vi "piecyk_23.vi"(3 "Stop Button":bool, 4 "Desired Temperature °C":i32(knob) min=-20 max=50 step=1 scale=-20.0..50.0, 5 "VISA resource":refnum<visa-resource-name>) -> (0 "Heating ON/OFF":bool, 1 "Temp. Chart":i32(graph), 2 "Current temp °C":dbl(slide) scale=-20.0..50.0 scale format="%#_1p")   [LabVIEW 2024]
doc: "Use this template to build a standard state machine design pattern. Each state executes code and determines which state to transition to. Contrast this design pattern with the User Interface Event Handler pattern, in which code executes in response to user actions. Contrast this design pattern also with the Queued Message Handler pattern, in which each message handling code can queue zero or more new messages.\nNote: This template does not contain the most recent programming guidelines recommended by National Instruments. For a complete, project-based implementation of the Standard State Machine pattern, use the Create Project dialog box instead of this template."
uses:
  piecyk.ctl
  <vilib>/Instr/_visa.llb/VISA Configure Serial Port (Instr).vi
panel:
  out "Temp indicator":string
  # "Time"
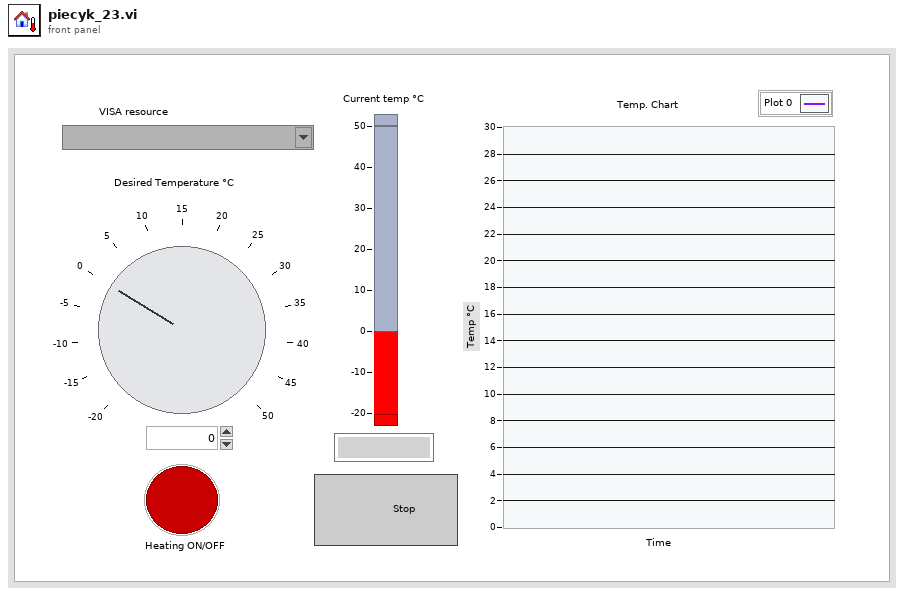
[diagram p1: front panel]
types:
  T1 = typedef "piecyk.ctl" = enum16{"Initialize", "Heating", "Ho Heating", "Stop"}
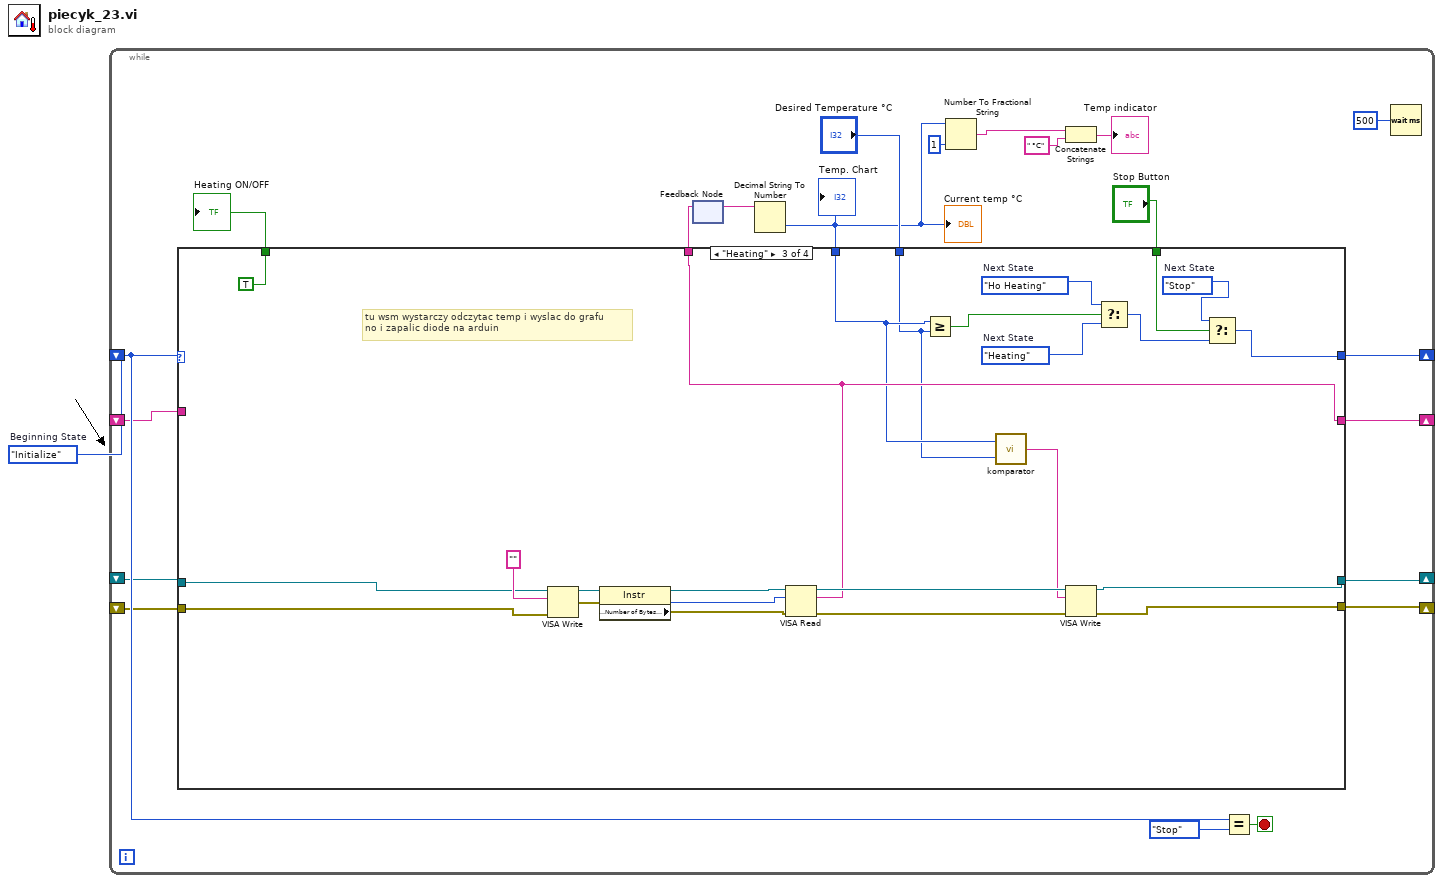
[diagram p0: block diagram]
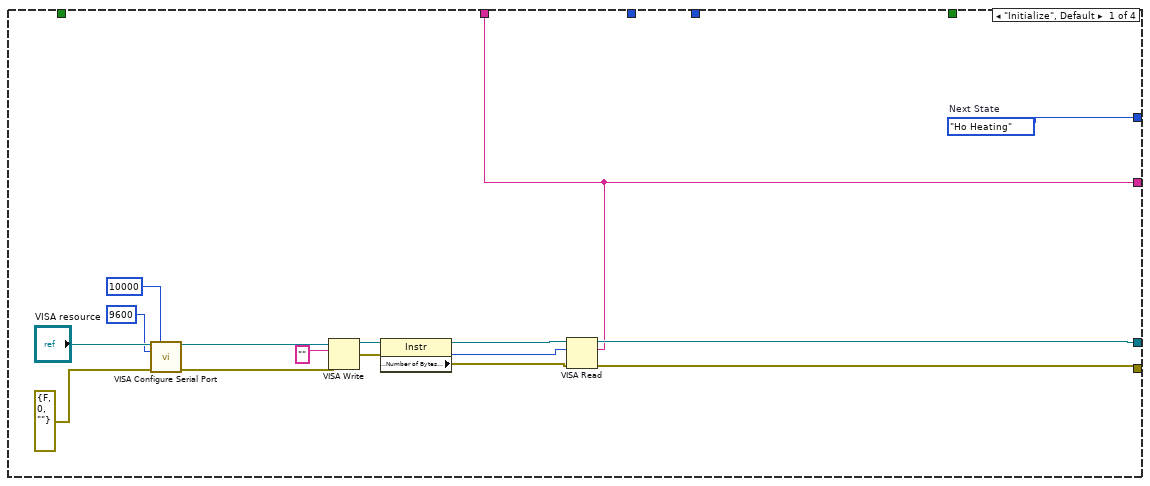
[diagram p2: hidden frame]
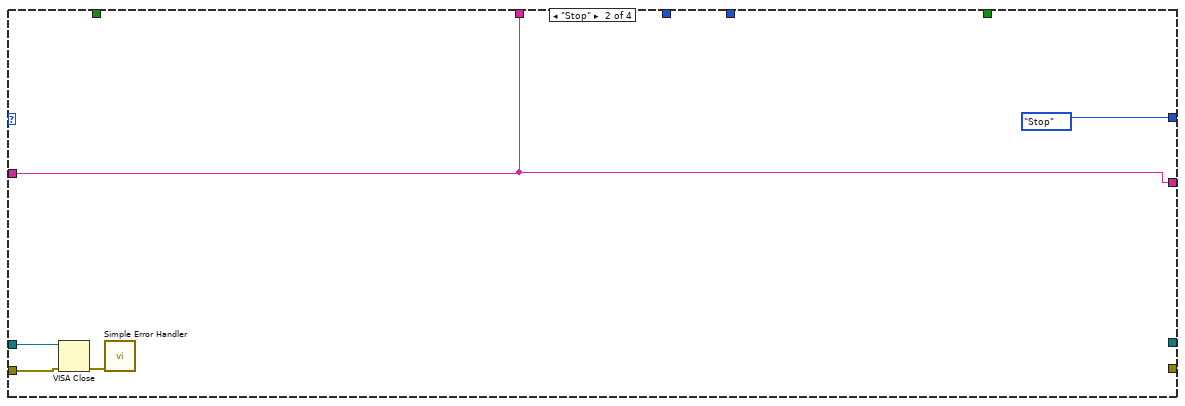
[diagram p3: hidden frame]
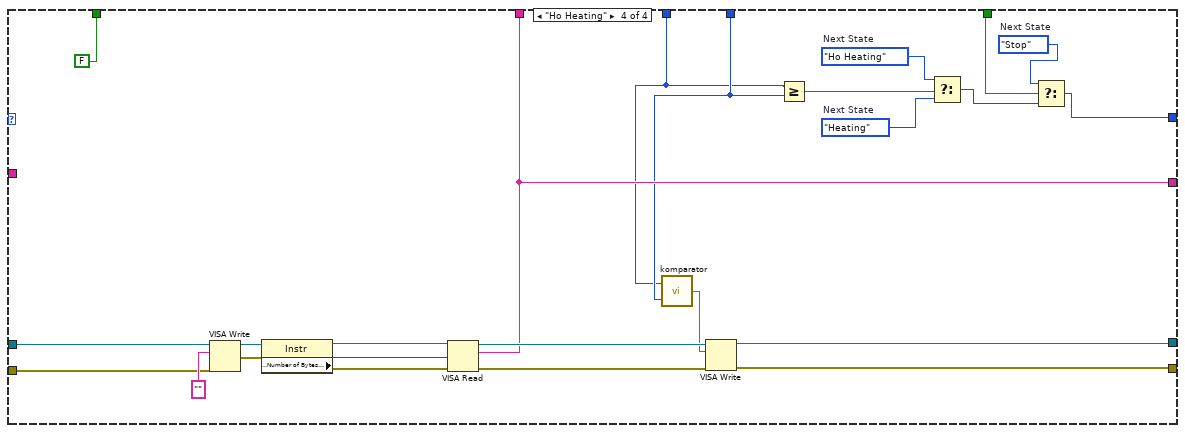
[diagram p4: hidden frame]
diagram:
  w1 = piecyk."Initialize"  # Beginning State
  n1 = while {
    shift-right: [w18] -> _
    shift-left: w1 -> [w20]
    shift-right: [w17] -> _
    shift-left: _ -> [w7]
    shift-right: [w16] -> _
    shift-left: _ -> [w6]
    shift-right: [w3] -> _
    shift-left: _ -> [w2]
    stop <- w22 stop-if-true
    n2 = feedback #1() -> (w5:string)  [unwired: 1 in]
    n3 = Decimal String To Number(string=w5) -> (number=w8:i32)  [unwired: 2 in, 1 out]
    "Temp. Chart" <- w8
    "Current temp °C" <- w8
    n4 = case shown="\"Heating\"" w20 {
      tunnel: [w36 piecyk."Stop" ("Next State") w62 w85] -> w18
      tunnel: w6 -> [_ w40 w54 w78]
      tunnel: w7 -> [_ w41 w53 w77]
      tunnel: [w25 _ w49 w73] -> w17
      tunnel: [w24 _ w50 w74] -> w16
      tunnel: "Desired Temperature °C" -> [_ _ w45 w70]
      tunnel: w8 -> [_ _ w46 w69]
      tunnel: [_ _ TRUE FALSE] -> w14
      tunnel: "Stop Button" -> [_ _ w65 w86]
      tunnel: [w23 w39 w47 w71] -> w4
      tunnel: [w23 w39 w47 w71] -> w3
      tunnel: w2 -> [_ w39 _ _]
      frame "Initialize", Default {
        w36 = piecyk."Ho Heating"  # Next State
        n5 = call-poly "VISA Configure Serial Port"("VISA resource name"="VISA resource", "timeout (10sec)"=u32 10000, "baud rate (9600)"=u32 9600, "error in (no error)"=errorcluster {"status"=FALSE, "code"=0, "source"=""} ("error in")) -> ("VISA resource name out"=w27:refnum<visa-resource-name>, "error out"=w26:errorcluster)  [unwired: 10 in]
        n6 = VISA Write(VISA resource name=w27, write buffer="", error in (no error)=w26) -> (VISA resource name out=w33:refnum<visa-resource-name>, error out=w32:errorcluster)  [unwired: 1 out]
        n7 = property class="Instr"(reference=w33, error in=w32) -> (reference out=w31:refnum<visa-resource-name>, error out=w30:errorcluster, "Serial Settings:Number of Bytes at Serial Port"=w29:u32)
        n8 = VISA Read(VISA resource name=w31, byte count=w29, error in (no error)=w30) -> (VISA resource name out=w24:refnum<visa-resource-name>, read buffer=w23:string, error out=w25:errorcluster)  [unwired: 1 out]
      }
      frame "Stop" {
        n9 = VISA Close(VISA resource name=w40, error in (no error)=w41) -> (error out=w42:errorcluster)
        n10 = call <vilib>:"Simple Error Handler.vi"("error in (no error)"=w42) -> ()  [unwired: 4 in, 5 out]
      }
      frame "Heating" {
        w64 = piecyk."Stop"  # Next State
        w67 = piecyk."Heating"  # Next State
        w66 = piecyk."Ho Heating"  # Next State
        # "tu wsm wystarczy odczytac temp i wyslac do grafu\nno i zapalic diode na arduin"
        n11 = VISA Write(VISA resource name=w54, write buffer="", error in (no error)=w53) -> (VISA resource name out=w60:refnum<visa-resource-name>, error out=w59:errorcluster)  [unwired: 1 out]
        n12 = property class="Instr"(reference=w60, error in=w59) -> (reference out=w58:refnum<visa-resource-name>, error out=w57:errorcluster, "Serial Settings:Number of Bytes at Serial Port"=w56:u32)
        n13 = VISA Read(VISA resource name=w58, byte count=w56, error in (no error)=w57) -> (VISA resource name out=w52:refnum<visa-resource-name>, read buffer=w47:string, error out=w51:errorcluster)  [unwired: 1 out]
        n14 = Greater Or Equal?(x=w46, y=w45) -> (x >= y?=w44:bool)
        n15 = call "komparator.vi"("Docelowa"=w45, "Aktualna"=w46) -> ("Output"=w48:string)
        n16 = VISA Write(VISA resource name=w52, write buffer=w48, error in (no error)=w51) -> (VISA resource name out=w50:refnum<visa-resource-name>, error out=w49:errorcluster)  [unwired: 1 out]
        n17 = Select(t=w66, s=w44, f=w67) -> (s? t:f=w63:T1)
        n18 = Select(t=w64, s=w65, f=w63) -> (s? t:f=w62:T1)
      }
      frame "Ho Heating" {
        w88 = piecyk."Stop"  # Next State
        w90 = piecyk."Heating"  # Next State
        w89 = piecyk."Ho Heating"  # Next State
        n19 = VISA Write(VISA resource name=w78, write buffer="", error in (no error)=w77) -> (VISA resource name out=w84:refnum<visa-resource-name>, error out=w83:errorcluster)  [unwired: 1 out]
        n20 = property class="Instr"(reference=w84, error in=w83) -> (reference out=w82:refnum<visa-resource-name>, error out=w81:errorcluster, "Serial Settings:Number of Bytes at Serial Port"=w80:u32)
        n21 = VISA Read(VISA resource name=w82, byte count=w80, error in (no error)=w81) -> (VISA resource name out=w76:refnum<visa-resource-name>, read buffer=w71:string, error out=w75:errorcluster)  [unwired: 1 out]
        n22 = call "komparator.vi"("Docelowa"=w70, "Aktualna"=w69) -> ("Output"=w72:string)
        n23 = VISA Write(VISA resource name=w76, write buffer=w72, error in (no error)=w75) -> (VISA resource name out=w74:refnum<visa-resource-name>, error out=w73:errorcluster)  [unwired: 1 out]
        n24 = Greater Or Equal?(x=w69, y=w70) -> (x >= y?=w68:bool)
        n25 = Select(t=w89, s=w68, f=w90) -> (s? t:f=w87:T1)
        n26 = Select(t=w88, s=w86, f=w87) -> (s? t:f=w85:T1)
      }
    }
    "Heating ON/OFF" <- w14
    n27 = feedback-in #1(w4) -> ()
    n28 = Number To Fractional String(number=w8, precision (6)=i16 1) -> (F-format string=w11:string)  [unwired: 2 in]
    n29 = Concatenate Strings(w11, " °C") -> (→"Temp indicator":string)
    n30 = Equal?(x=w20, y=piecyk."Stop" ("States")) -> (x = y?=w22:bool)
    n31 = Wait (ms)(milliseconds to wait=u32 500) -> ()  [unwired: 1 out]
  }
